vi "Launcher.vi"() -> ()   [LabVIEW 2015]
uses:
  ISA010_module/ISA010_module.lvlib
panel:
  in  "String":string
  # "ISA010V GATEWAY"
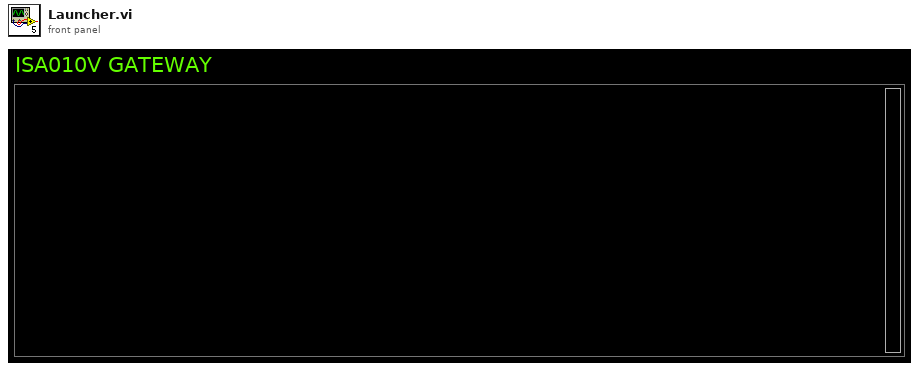
[diagram p1: front panel]
types:
  T1 = typedef "ISA010_module.lvlib/Broadcast Events--cluster.ctl" = cluster{"Module Did Init":refnum<user-event>, "Status Updated":refnum<user-event>, "Error Reported":refnum<user-event>, "Module Did Stop":refnum<user-event>, "Update Module Execution Status":refnum<user-event>, "ISA010State":refnum<user-event>}
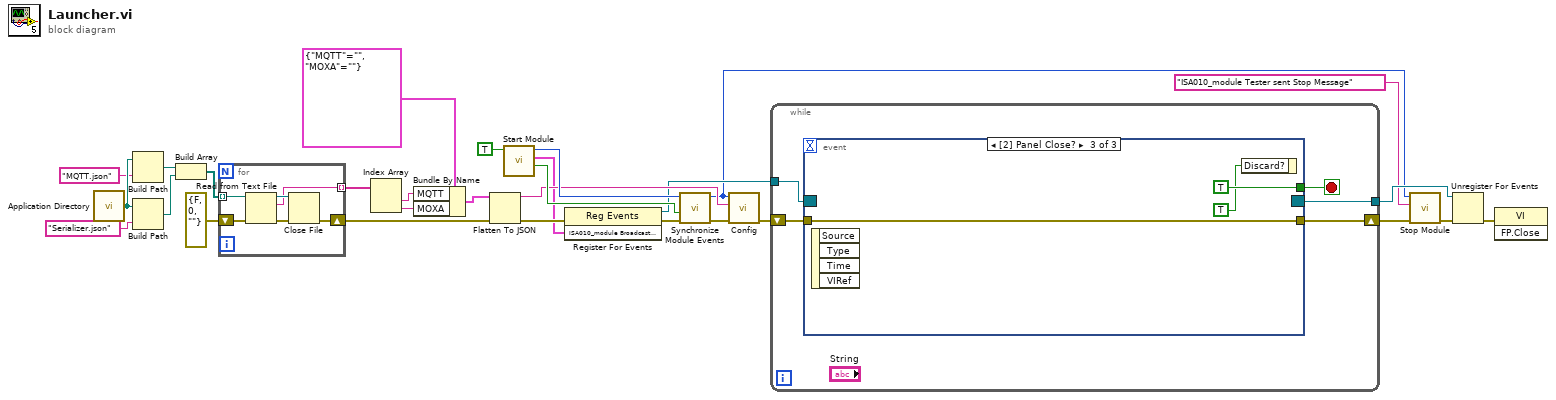
[diagram p0: block diagram]
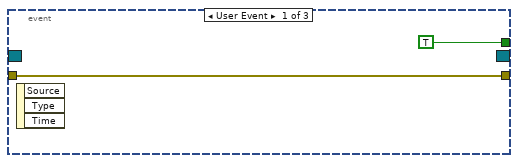
[diagram p2: hidden frame]
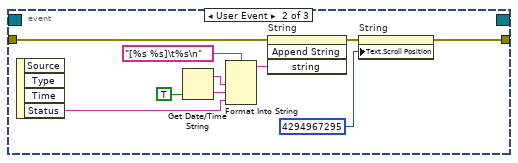
[diagram p3: hidden frame]
diagram:
  n1 = call <vilib>:"Application Directory.vi"() -> ("Application Directory"=w29:path)
  n2 = Build Path(base path=w29, name or relative path="MQTT.json") -> (appended path=w27:path)
  n3 = Build Path(base path=w29, name or relative path="Serializer.json") -> (appended path=w28:path)
  n4 = Build Array(w27, w28) -> (w26:path[])
  n5 = for {
    tunnel: w26 -> [w32] mode=indexing
    tunnel: [w33] -> w24 mode=indexing
    shift-right: [w31] -> w17
    shift-left: errorcluster {"status"=FALSE, "code"=0, "source"=""} ("error out") -> [w30]
    n6 = Read from Text File(file (use dialog)=w32, error in=w30) -> (refnum out=w34:refnum<file>, text=w33:string, error out=w35:errorcluster)  [unwired: 2 in, 1 out]
    n7 = Close File(refnum=w34, error in=w35) -> (error out=w31:errorcluster)  [unwired: 1 out]
  }
  n8 = Index Array(array=w24) -> (element #1=w20:string, element #2=w19:string)  [unwired: 2 in]
  n9 = Bundle By Name(cluster=cluster{"MQTT":string, "MOXA":string} {"MQTT"="", "MOXA"=""}, "MQTT"=w20, "MOXA"=w19) -> (w18:cluster{"MQTT":string, "MOXA":string})
  n10 = Flatten To JSON(anything=w18, error in (no error)=w17) -> (JSON string=w13:string, 11:w11:errorcluster)  [unwired: 1 in]
  n11 = call "Start Module.vi"("Run as Singleton? (F)"=TRUE) -> ("Wait for Event Sync?"=w16:bool, "ISA010_module Broadcast Events"=w10:T1, "Module ID"=w15:i32)  [unwired: 7 in, 1 out]
  n12 = register-events(error in=w11, w10) -> (reference out=w7:refnum<event-registration>, error out=w9:errorcluster)  [unwired: 1 in]
  n13 = call "Synchronize Module Events.vi"("error in (no error)"=w9, "Wait for Event Sync?"=w16, "Module ID"=w15) -> ("error out"=w12:errorcluster, "Module ID (dup)"=w4:i32)  [unwired: 7 in]
  n14 = call "Config.vi"("error in (no error)"=w12, "ConfigJson"=w13, "Module ID"=w4) -> ("error out"=w8:errorcluster)  [unwired: 8 in]
  n15 = while {
    tunnel: w7 -> [w40]
    shift-right: [w39] -> w3
    shift-left: w8 -> [w38]
    tunnel: [w37] -> w6
    stop <- w36 stop-if-true
    n16 = event shown="[2] Panel Close?" {
      selector: w40 -> [_ _ _]
      dyn-events: [_ _ _] -> w37
      timeout: _ -> [_ _ _]
      tunnel: [w42 w44 w53] -> w39
      tunnel: w38 -> [w42 w52 w53]
      tunnel: [TRUE _ TRUE] -> w36
      event User Event {
        n17 = event-data() -> ()  [unwired: 1 in, 3 out]
      }
      event User Event {
        n18 = event-data() -> ("Status"=w47:string)  [unwired: 1 in, 3 out]
        n19 = Get Date/Time String(want seconds? (F)=TRUE) -> (date string=w49:string, time string=w48:string)  [unwired: 2 in]
        n20 = Format Into String(format string="[%s %s]\t%s\n", w49, w48, w47) -> (resulting string=w46:string)  [unwired: 2 in, 1 out]
        n21 = invoke on="String" class="Str" method="Append String"(error in=w52, "string"=w46) -> (error out=w45:errorcluster)  [unwired: 2 in, 3 out]
        n22 = property on="String" class="Str"(error in=w45, "Text.Scroll Position"=u32 4294967295) -> (error out=w44:errorcluster)  [unwired: 1 in, 1 out]
      }
      event Panel Close? {
        n23 = event-data() -> ()  [unwired: 1 in, 4 out]
        n24 = event-data("Discard?"=TRUE) -> ()  [unwired: 1 in, 1 out]
      }
    }
  }
  n25 = call "Stop Module.vi"("error in (no error)"=w3, "Origin"="ISA010_module Tester sent Stop Message", "Module ID"=w4) -> ("error out"=w2:errorcluster)  [unwired: 8 in]
  n26 = Unregister For Events(event registration refnum=w6, error in=w2) -> (error out=w1:errorcluster)
  n27 = invoke class="VI" method="FP.Close"(error in=w1) -> ()  [unwired: 2 in, 3 out]
